vi "Set Internal Tv.vi"(6 "parseError? T:Yes":bool=TRUE, 8 "error in (no error)":errorcluster, 10 "Tv (0s)":u16 max=999, 11 "VISA resource name":refnum<visa-resource-name>) -> (0 "error out":errorcluster, 3 "VISA resource name out":refnum<visa-resource-name>)   [LabVIEW 2018, in "JULABO DeviceDriver.lvlib"]
doc: "This VI adjusts the Lead time <B>Tv</B> (Differential component) in case of internal temperature control.\n\nThe differential component reduces the control settling time. An insufficient lead time will prolong the time required to compensate for disturbance effects and cause high overshoot during run-up. An excessive lead time could cause instabilities (oscillations) to occur.\nAdjustable range: <B>0 ... 999</B>"
uses:
  JULABO DeviceDriver.lvlib
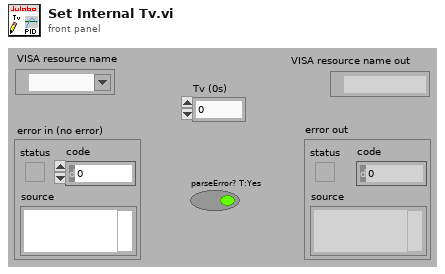
[diagram p1: front panel]
types:
  T1 = typedef "JULABO DeviceDriver.lvlib/InstrumentType.ctl" = enum8{"Default", "FC-Series", "HT30/HT60", "LC4"}
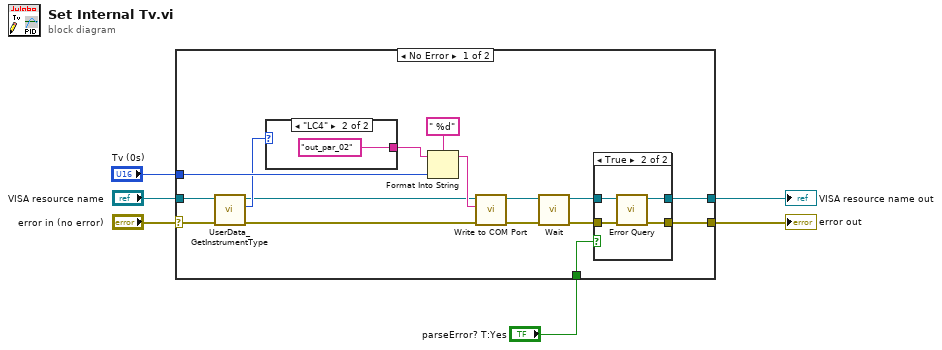
[diagram p0: block diagram]
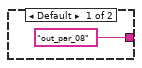
[diagram p2: hidden frame]
diagram:
  n1 = case shown="No Error" "error in (no error)" {
    selector: "error in (no error)" -> [w10 w31]
    tunnel: "VISA resource name" -> [w11 w32]
    tunnel: [w21 w31] -> w5
    tunnel: [w20 w32] -> w4
    tunnel: "Tv (0s)" -> [w22 _]
    tunnel: "parseError? T:Yes" -> [w19 _]
    frame No Error {
      n2 = call "UserData_GetInstrumentType.vi"("Fehler (Eingang)"=w10, "VISA resource name in"=w11) -> ("Fehler (Ausgang)"=w8:errorcluster, "InstrumentType"=w12:T1, "VISA resource name out"=w9:refnum<visa-resource-name>)  [unwired: 3 in]
      n3 = case shown="\"LC4\"" w12 {
        tunnel: ["out_par_08" "out_par_02"] -> w7
        frame Default {
        }
        frame "LC4" {
        }
      }
      n4 = Format Into String(format string=" %d", initial string=w7, w22) -> (resulting string=w13:string)  [unwired: 1 in, 1 out]
      n5 = call "Write to COM Port.vi"("error in"=w8, "Command (input)"=w13, "VISA resource name in"=w9) -> ("error out"=w17:errorcluster, "VISA resource name out"=w18:refnum<visa-resource-name>)  [unwired: 7 in]
      n6 = call "Wait.vi"("error in"=w17, "VISA resource name in"=w18) -> ("error out"=w15:errorcluster, "VISA resource name out"=w16:refnum<visa-resource-name>)  [unwired: 4 in]
      n7 = case shown="True" w19 {
        tunnel: w16 -> [w26 w30]
        tunnel: w15 -> [w25 w29]
        tunnel: [w26 w28] -> w20
        tunnel: [w25 w27] -> w21
        frame False {
        }
        frame True {
          n8 = call "Error Query.vi"("error in (no error)"=w29, "VISA resource name"=w30) -> ("error out"=w27:errorcluster, "VISA resource name out"=w28:refnum<visa-resource-name>)  [unwired: 6 in, 2 out]
        }
      }
    }
    frame Error {
    }
  }
  "error out" <- w5
  "VISA resource name out" <- w4
